vi "系统设置.vi"() -> ()   [LabVIEW 2016]
uses:
  <vilib>/Utility/miscctls.llb/LVPointTypeDef.ctl
  <vilib>/ptbypt/NI_PtbyPt.lvlib
  <vilib>/Utility/config.llb/NI_LVConfig.lvlib
  PLC/PLC.lvlib
panel:
  in  "updateconfiguration":T1={"主机"="27.154.58.30", "用户"="update", "密码"="std23506", "远程路径"="数据传输系统\\平台数据传输系统.exe", "下载文件名"="平台数据传输系统.exe", "软件版本"=""}
  in  "周期运行启动参数":T2
  in  "超标浓度报警":bool
  in  "更新":bool
  in  "模块启用配置":bool
  in  "短信报警设置":bool
  in  "首页显示设置":bool
  in  "跨度核查":bool
  in  "空白核查":bool
  out "选项卡控件":enum32{"自由设定", "国标协议", "流量设定"}(tab)
  in  "24H周期设置":bool[](xcontrol)
  in  "运行间隔":i16=4 min=1 max=24
  in  "流量阈值":dbl=4.0 min=1.0 max=24.0
  in  "时间阈值":u16=4 min=1 max=24
  in  "周期设置":enum16{"自由设定", "国标协议", "流量设定"}(ring)
  out "x = y?":bool
  in  "质控启动日期":string(combo)="关闭"
  in  "跨度核查时间":T3(ring)=enum."06H"
  in  "空白核查时间":T3(ring)=enum."02H"
  in  "输入密码":dbl
  out "布尔":bool
  in  "副屏显示设置":bool
  in  "开机启动":bool caption="氨氮禁用"
  in  "运行模式":enum16{"维护模式", "常规模式", "应急模式", "质控模式"}(ring)
  # "注：周期设置分为自由设定和国标协议两种。\n1：选择自由设定情况下：运行间隔将不可选用并变灰色，周期设置可自由手动勾选\n2：选择国标协议情况下：周期时间将由运行间隔选择的时间决定，下方周期设置被禁用并无法手动勾选。\n3：选择流量设定情况下：瞬时流量连续超过流量阈值到达时间阈值设定值，仪器将自动开启测量。"
  # "质控频次："
  # "零点核查时间："
  # "跨度核查时间："
  # "启动周期设置"
  # "m3/S"
  # "秒"
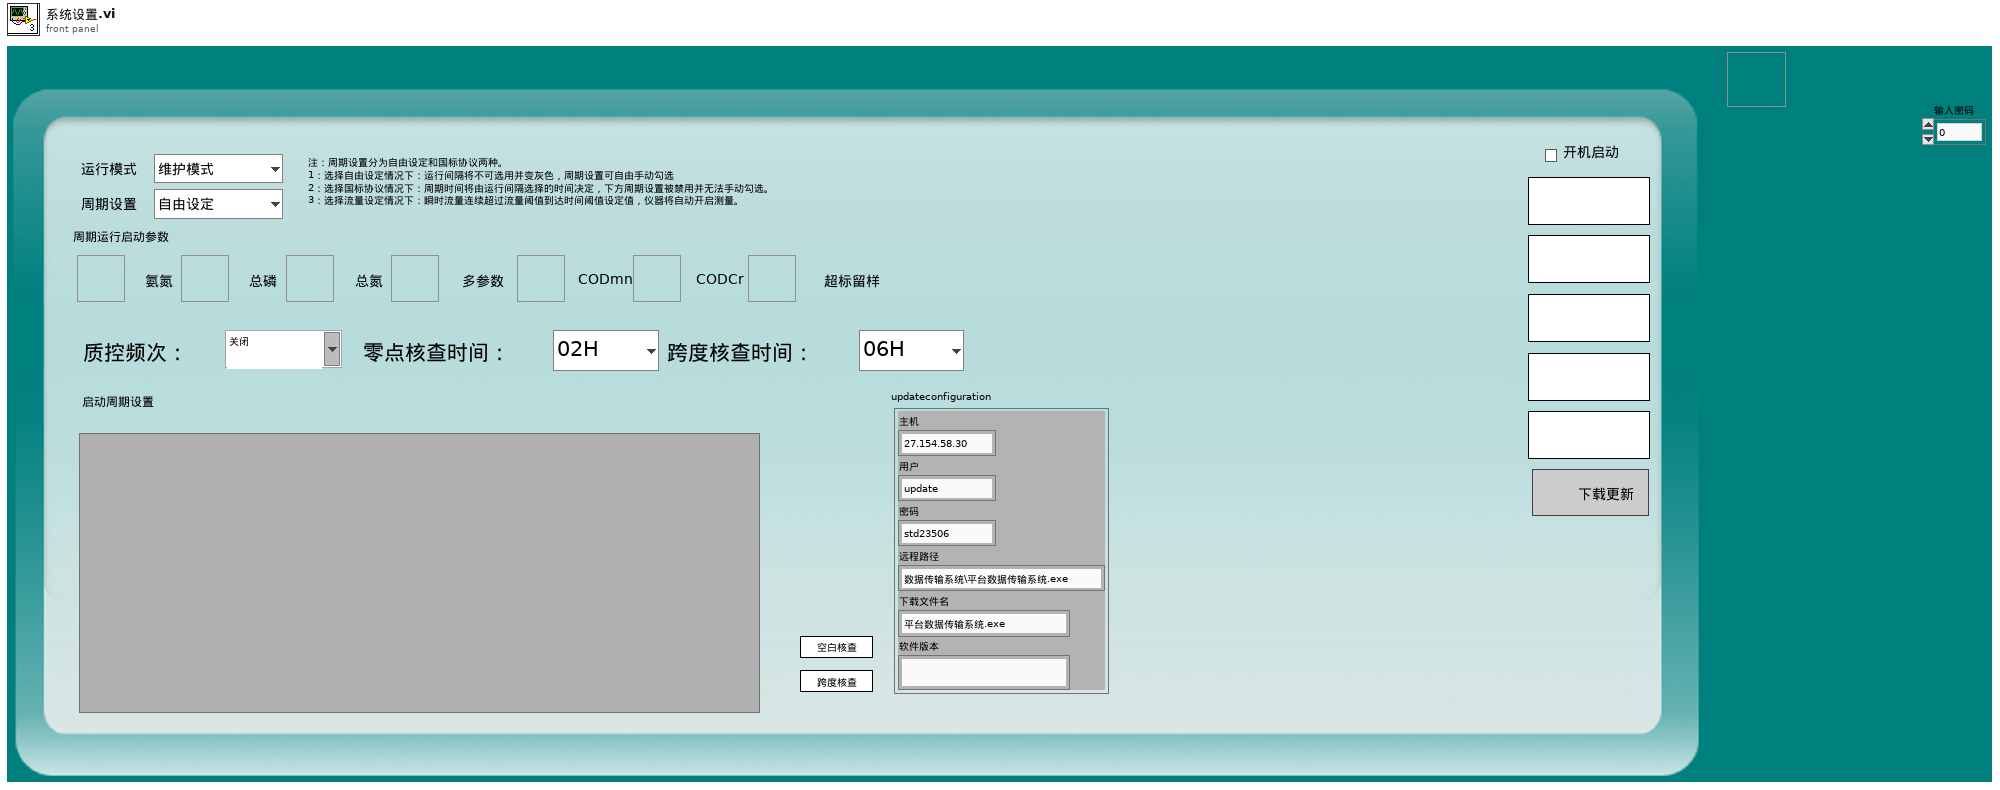
[diagram p1: front panel]
types:
  T1 = cluster{"主机":string, "用户":string, "密码":string, "远程路径":string, "下载文件名":string, "软件版本":string}
  T2 = cluster{"氨氮":bool, "总磷":bool, "总氮":bool, "多参数":bool, "CODmn":bool, "CODCr":bool, "超标留样":bool}
  T3 = enum16{"00H", "01H", "02H", "03H", "04H", "05H", "06H", "07H", "08H", "09H", "10H", "11H", "12H", "13H", "14H", "15H", "16H", "17H", "18H", "19H", "20H", "21H", "22H", "23H", "关闭"}
  T4 = typedef "NI_LVConfig.lvlib/Config Data RefNum.ctl" = refnum<k1>
  T5 = typedef "LVPointTypeDef.ctl" = cluster{"Horizontal":i16, "Vertical":i16}
  T6 = enum32{"Bad", "Idle", "Run top level", "Running"}
  T7 = enum32{"Invalid", "Standard", "Closed", "Hidden", "Minimized", "Maximized"}
  T8 = cluster{"运行模式":enum16{"维护模式", "常规模式", "应急模式", "质控模式"}}
  T9 = enum16{"启动测量", "标样核查", "零点核查", "跨度核查", "空白测试", "平行样测试", "加标回收", "空白校准", "标样校准", "初始化（清洗）", "停止测试", "仪器重启", "校时", "模式设置", "测量间隔设置"}
  T10 = cluster{"测量模式":enum16{"水样测量", "标样核查", "零点核查", "跨度核查", "空白测试", "加标回收", "平行样", "校零", "校标"}}
  T11 = cluster{"测试模式":enum16{"正常测试", "集成干预", "加标回收"}, "参数启用":cluster{"氨氮":bool, "总磷":bool, "总氮":bool, "多参数":bool, "CODMn":bool, "CODcr":bool, "超标留样":bool}}
  T12 = cluster{"运行模式":enum16{"维护模式", "常规模式", "应急模式", "质控模式"}, "质控频次":enum16{"关闭", "每天", "星期一", "星期二", "星期三", "星期四", "星期五", "星期六", "星期日"}, "空白核查时间":u16, "跨度核查时间":u16, "24H周期设置":bool[]}
  T13 = typedef "LVDateTimeRec.ctl" = cluster{"秒数的小数部分":dbl, "秒":i32, "分":i32, "时":i32, "日":i32, "月":i32, "年":i32, "天数（周）":i32, "天数（年）":i32, "DST":i32}
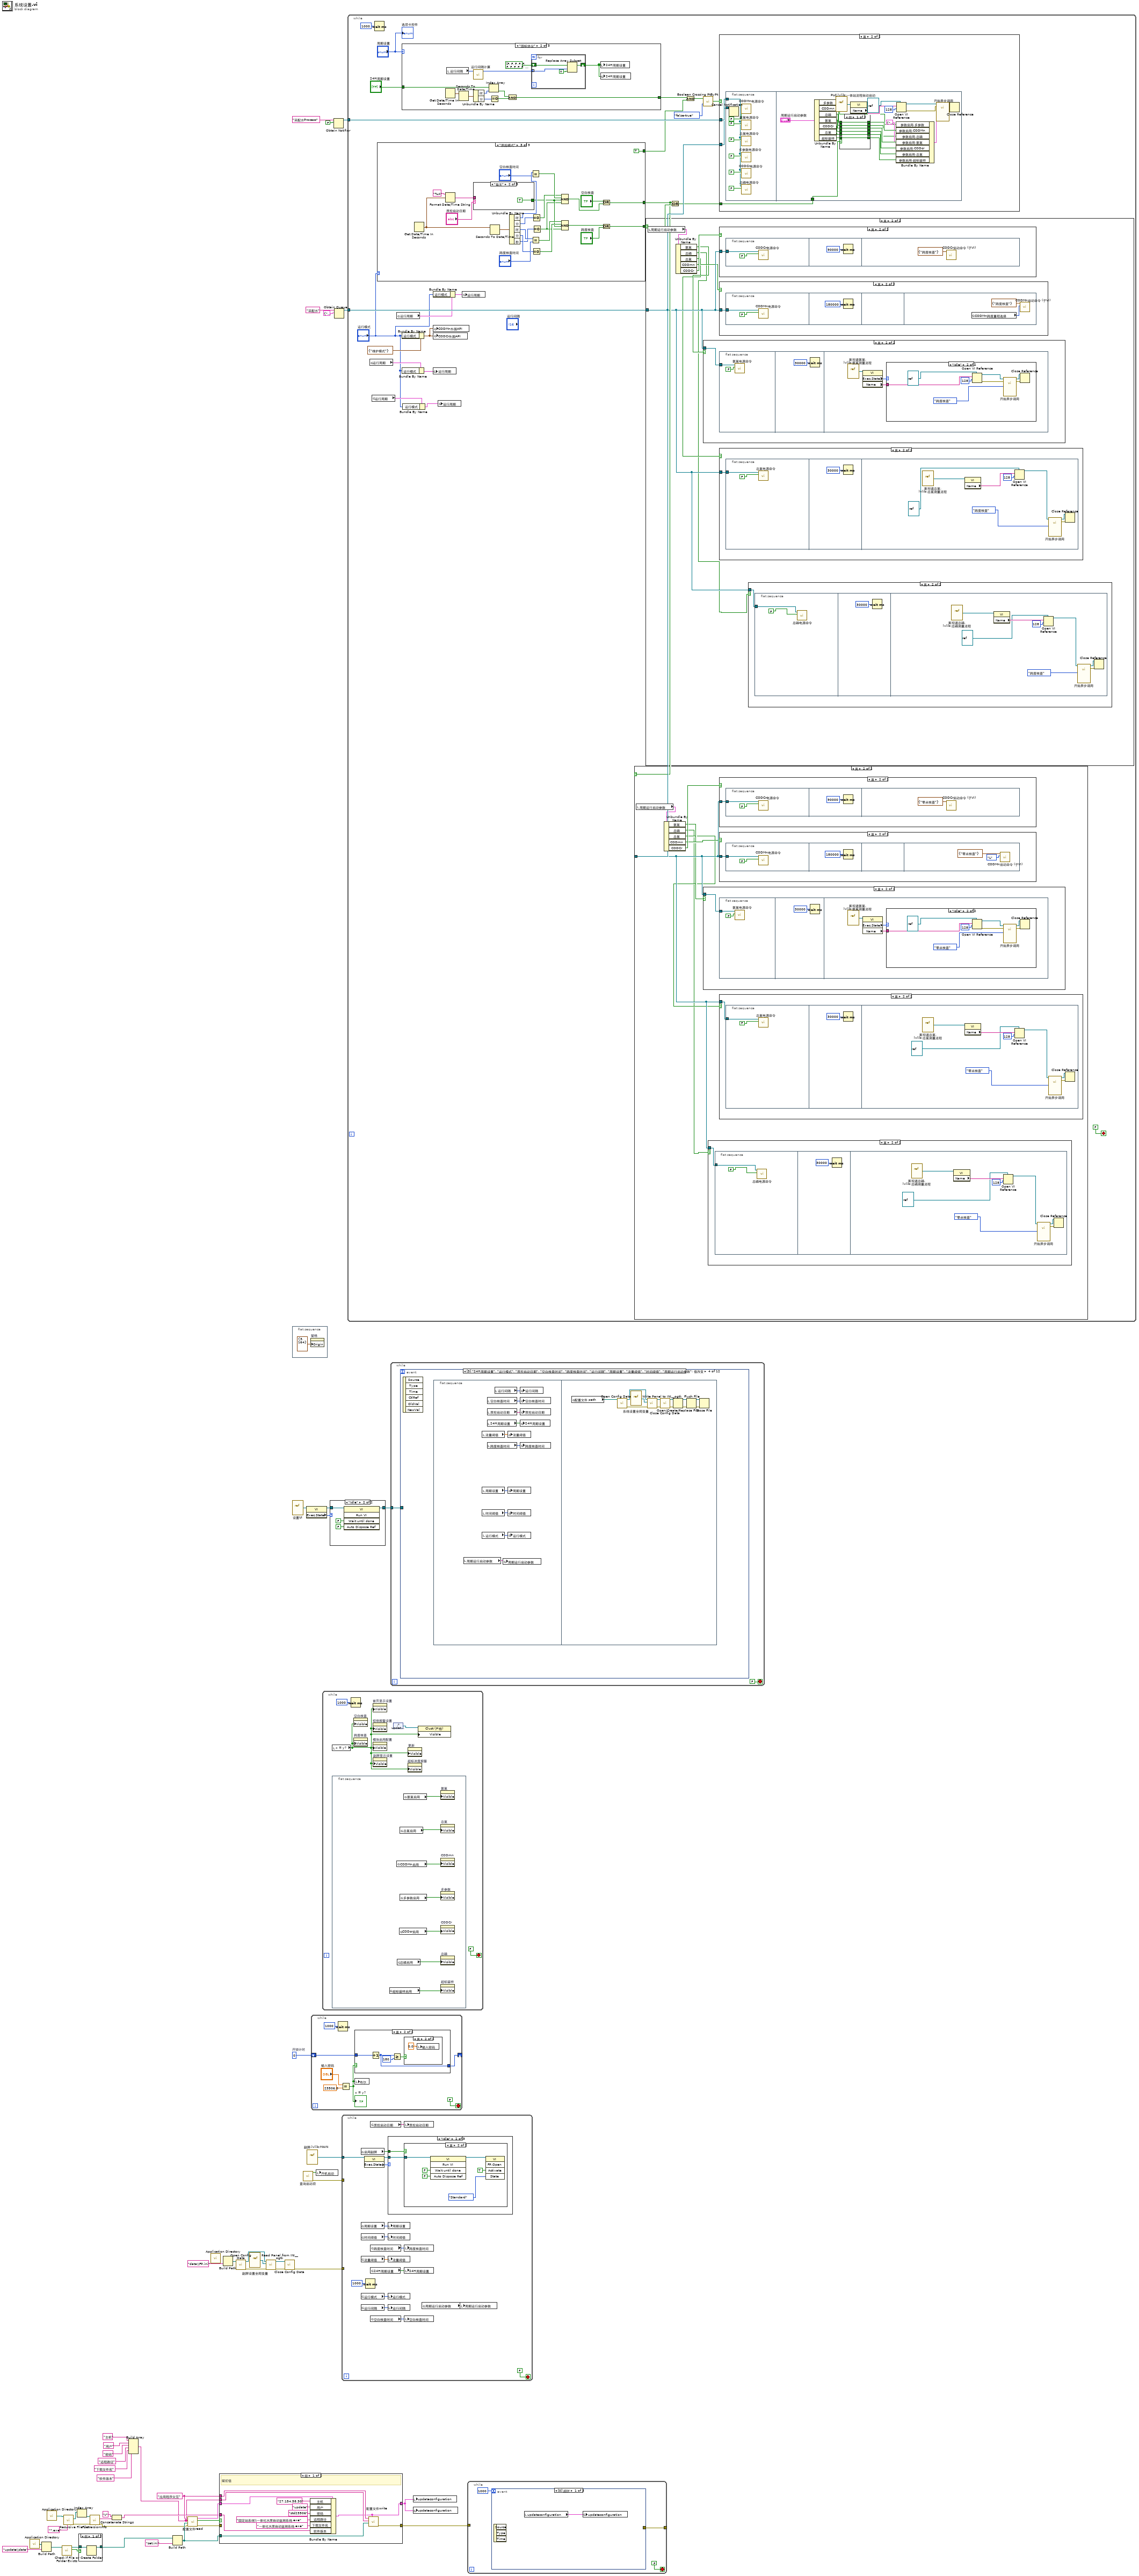
[diagram p0: block diagram]
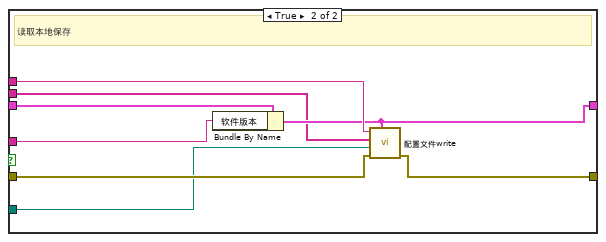
[diagram p3: hidden frame]
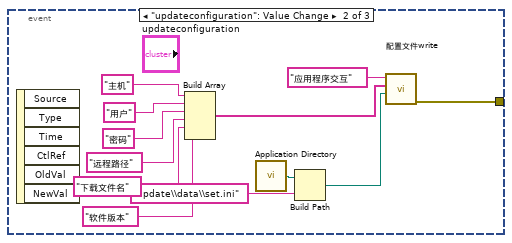
[diagram p4: hidden frame]
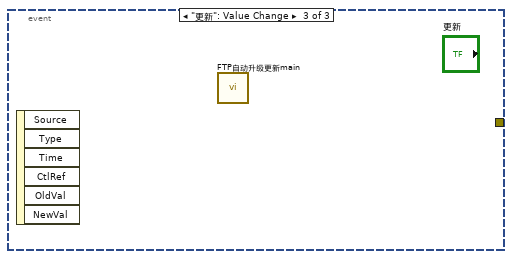
[diagram p5: hidden frame]
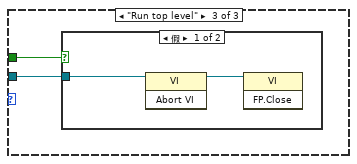
[diagram p11: hidden frame]
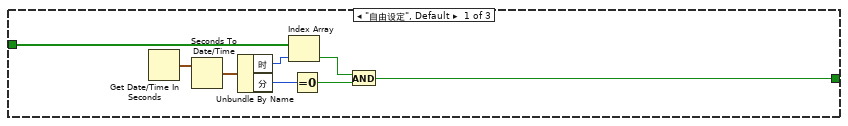
[diagram p13: hidden frame]
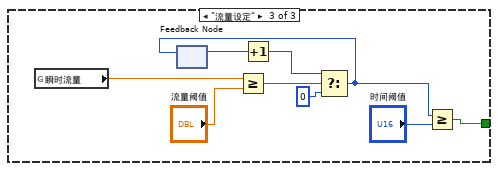
[diagram p14: hidden frame]
diagram:
  w28 = "应用程序交互" ("section")
  w48 = u32 0  # 开锁计时
  n1 = call <vilib>:"Application Directory.vi"() -> ("Application Directory"=w5:path)
  n2 = Build Path(base path=w5, name or relative path="update\\data" ("名称或相对路径")) -> (appended path=w6:path)
  n3 = call <vilib>:"Application Directory.vi"() -> ("Application Directory"=w23:path)
  n4 = call <vilib>:"Check if File or Folder Exists.vi"("path"=w6) -> ("file or folder exists?"=w7:bool, "dup path"=w8:path)  [unwired: 8 in, 1 out]
  n5 = call <vilib>:"Recursive File List.vi"("pattern"="*.exe", "Folder Path"=w23) -> ("error out"=w20:errorcluster, "All Files in Dir"=w22:path[])  [unwired: 5 in, 3 out]
  n6 = Index Array(array=w22) -> (element=w24:path)  [unwired: 1 in]
  n7 = case shown="假" w7 {
    tunnel: w8 -> [w54 w55]
    tunnel: [w53 w55] -> w3
    frame False {
      n8 = Create Folder(path (use dialog)=w54) -> (created path=w53:path)  [unwired: 2 in, 2 out]
    }
    frame True {
    }
  }
  n9 = call <vilib>:"FileVersionInfo.vi"("error in (no error)"=w20, "Application Path in"=w24) -> ("error out"=w17:errorcluster, "File Version Info"=w18:string)  [unwired: 6 in, 2 out]
  n10 = Concatenate Strings("V" ("字符串"), w18) -> (w16:string)
  n11 = Build Array("主机" ("section"), "用户" ("section"), "密码" ("key"), "远程路径" ("key"), "下载文件名" ("key"), "软件版本" ("key")) -> (w2:string[])
  n12 = Build Path(base path=w3, name or relative path="set.ini" ("名称或相对路径")) -> (appended path=w27:path)
  n13 = call "配置文件read.vi"("error in (no error)"=w17, "configuration file path"=w27, "键数组"=w2, "段"=w28) -> ("error out"=w26:errorcluster, "section exists?"=w29:bool, "updateconfiguration"=w25:T1)  [unwired: 5 in]
  n14 = call <vilib>:"Application Directory.vi"() -> ()  [unwired: 1 out]
  n15 = case shown="假" w29 {
    tunnel: w2 -> [w67 w71]
    tunnel: w28 -> [w66 w75]
    tunnel: w27 -> [w65 w69]
    tunnel: w26 -> [_ w70]
    tunnel: [w64 w68] -> w15
    tunnel: w25 -> [w58 w74]
    tunnel: [w56 w72] -> w1
    tunnel: w16 -> [w57 w73]
    frame False {
      # "赋初值"
      n16 = Bundle By Name(cluster=w58, "主机"="27.154.58.30" ("key"), "用户"="update", "密码"="std23506", "远程路径"="固定站系统\\一体化水质自动监测系统.exe", "下载文件名"="一体化水质自动监测系统.exe", "软件版本"=w57) -> (w56:T1)
      n17 = call "配置文件write.vi"("updateconfiguration"=w56, "configuration file path"=w65, "键数组"=w67, "段"=w66) -> ("error out"=w64:errorcluster)  [unwired: 7 in]
    }
    frame True {
      # "读取本地保存"
      n18 = Bundle By Name(cluster=w74, "软件版本"=w73) -> (w72:T1)
      n19 = call "配置文件write.vi"("updateconfiguration"=w72, "error in (no error)"=w70, "configuration file path"=w69, "键数组"=w71, "段"=w75) -> ("error out"=w68:errorcluster)  [unwired: 6 in]
    }
  }
  n20 = Build Path(name or relative path="data\\FP.ini" ("名称或相对路径")) -> (appended path=w37:path)  [unwired: 1 in]
  n21 = call <vilib>:"Open Config Data.vi"("configuration file path"=w37) -> ("error out"=w36:errorcluster, "refnum"=w33:T4)  [unwired: 8 in, 1 out]
  n22 = vi-ref "副屏设置全局变量.vi"() -> (w34:refnum<vi>)
  n23 = call <userlib>:"Read Panel from INI__ogtk.vi"("error in (no error)"=w36, "VI ref"=w34, "refnum"=w33) -> ("error out"=w35:errorcluster, "refnum out"=w32:T4)  [unwired: 7 in]
  n24 = call <vilib>:"Close Config Data.vi"("error in (no error)"=w35, "refnum"=w32) -> ("error out"=w31:errorcluster)  [unwired: 8 in, 1 out]
  n25 = flat-sequence {
    frame #0 {
      n26 = property on="窗格" class="Pane"("Origin"=T5 {"Horizontal"=3, "Vertical"=164} ("原点")) -> ()  [unwired: 2 in, 2 out]
    }
  }
  n27 = vi-ref "设置UI.vi"() -> (w43:refnum<vi>)
  n28 = call "查询启动项.vi"() -> ("error out"=w39:errorcluster, "包含启动项"=w49:bool)  [unwired: 9 in, 1 out]
  n29 = property class="VI"(reference=w43) -> (reference out=w41:refnum<vi>, "Exec.State"=w42:T6)  [unwired: 1 in, 1 out]
  n30 = vi-ref "副屏.lvlib:MAIN.vi"() -> (w44:refnum<vi>)
  n31 = while {
    shift-right: [w78] -> _
    shift-left: w48 -> [w79]
    stop <- FALSE stop-if-true
    n32 = Wait (ms)(milliseconds to wait=u32 1000 ("等待时间（毫秒）")) -> ()  [unwired: 1 out]
    n33 = Equal?(x="输入密码", y=23506.0) -> (x = y?=w77:bool)
    "x = y?" <- w77
    n34 = case shown="真" w77 {
      tunnel: w79 -> [_ w87]
      tunnel: [_ w86] -> w78
      frame False {
      }
      frame True {
        n35 = Increment(x=w87) -> (x+1=w86:u32)
        n36 = Greater Or Equal?(x=w86, y=u32 180) -> (x >= y?=w84:bool)
        n37 = case shown="真" w84 {
          frame False {
          }
          frame True {
            n38 = local write "输入密码"(0.0 ("输入密码")) -> ()
          }
        }
      }
    }
    n39 = local write "布尔"(w77) -> ()
  }
  n40 = local write "开机启动"(w49) -> ()
  n41 = while {
    stop <- FALSE stop-if-true
    n42 = local read "x = y?"() -> (w90:bool)
    n43 = flat-sequence {
      frame #0 {
        n44 = global read "系统设置全局变量.vi" "超标留样启用"() -> (w93:bool)
        n45 = global read "系统设置全局变量.vi" "CODMn启用"() -> (w97:bool)
        n46 = global read "系统设置全局变量.vi" "总磷启用"() -> (w94:bool)
        n47 = global read "系统设置全局变量.vi" "CODcr启用"() -> (w95:bool)
        n48 = global read "系统设置全局变量.vi" "总氮启用"() -> (w98:bool)
        n49 = global read "系统设置全局变量.vi" "多参数启用"() -> (w96:bool)
        n50 = global read "系统设置全局变量.vi" "氨氮启用"() -> (w99:bool)
        n51 = property on="氨氮" class="Bool (严格)"("Visible"=w99) -> ()  [unwired: 2 in, 2 out]
        n52 = property on="总氮" class="Bool (严格)"("Visible"=w98) -> ()  [unwired: 2 in, 2 out]
        n53 = property on="CODmn" class="Bool (严格)"("Visible"=w97) -> ()  [unwired: 2 in, 2 out]
        n54 = property on="多参数" class="Bool (严格)"("Visible"=w96) -> ()  [unwired: 2 in, 2 out]
        n55 = property on="CODCr" class="Bool (严格)"("Visible"=w95) -> ()  [unwired: 2 in, 2 out]
        n56 = property on="总磷" class="Bool (严格)"("Visible"=w94) -> ()  [unwired: 2 in, 2 out]
        n57 = property on="超标留样" class="Bool (严格)"("Visible"=w93) -> ()  [unwired: 2 in, 2 out]
      }
    }
    n58 = Wait (ms)(milliseconds to wait=u32 1000 ("等待时间（毫秒）")) -> ()  [unwired: 1 out]
    n59 = property on="空白核查" class="Bool"("Visible"=w90) -> ()  [unwired: 2 in, 2 out]
    n60 = property on="跨度核查" class="Bool"("Visible"=w90) -> ()  [unwired: 2 in, 2 out]
    n61 = property on="首页显示设置" class="Bool"("Visible"=w90) -> ()  [unwired: 2 in, 2 out]
    n62 = property on="短信报警设置" class="Bool"("Visible"=w90) -> ()  [unwired: 2 in, 2 out]
    n63 = property on="模块启用配置" class="Bool"("Visible"=w90) -> ()  [unwired: 2 in, 2 out]
    n64 = property on="副屏显示设置" class="Bool"("Visible"=w90) -> ()  [unwired: 2 in, 2 out]
    n65 = control-ref of="updateconfiguration"() -> (w89:refnum<vi>)
    n66 = property on="超标浓度报警" class="Bool"("Visible"=w90) -> ()  [unwired: 2 in, 2 out]
    n67 = property on="更新" class="Bool"("Visible"=w90) -> ()  [unwired: 2 in, 2 out]
    n68 = property class="Clust (严格)"(reference=w89, "Visible"=w90) -> ()  [unwired: 1 in, 2 out]
  }
  n69 = case shown="\"Idle\"" w42 {
    tunnel: w41 -> [w100 w104]
    tunnel: [w100 w103] -> w40
    frame "Bad", Default {
    }
    frame "Idle" {
      n70 = invoke class="VI" method="Run VI"(reference=w104, "Wait until done"=FALSE ("结束前等待"), "Auto Dispose Ref"=FALSE ("自动销毁引用")) -> (reference out=w103:refnum<vi>)  [unwired: 2 in, 4 out]
    }
  }
  n71 = Obtain Notifier(name (unnamed)="采配水Process" ("名称（未命名）"), notification data type=FALSE) -> (notifier out=w50:refnum<notifier>)  [unwired: 2 in, 2 out]
  n72 = Obtain Queue(name (unnamed)="采配水" ("名称（未命名）"), element data type=cluster{"命令":string, "数据":variant} {"命令"="", "数据"=variant}) -> (queue out=w45:refnum<queue>)  [unwired: 3 in, 2 out]
  n73 = while {
    tunnel: w44 -> [w117]
    tunnel: w39 -> [_]
    tunnel: w31 -> [_]
    stop <- FALSE stop-if-true
    n74 = global read "副屏设置全局变量.vi" "启用副屏"() -> (w115:bool)
    n75 = global read "系统设置全局变量.vi" "周期设置"() -> (w110:enum16{"自由设定", "国标协议", "流量设定"})
    n76 = global read "系统设置全局变量.vi" "时间阈值"() -> (w106:u16)
    n77 = global read "系统设置全局变量.vi" "流量阈值"() -> (w107:dbl)
    n78 = global read "系统设置全局变量.vi" "运行模式"() -> (w108:enum16{"维护模式", "常规模式", "应急模式", "质控模式"})
    n79 = global read "系统设置全局变量.vi" "运行间隔"() -> (w109:i16)
    n80 = property class="VI"(reference=w117) -> (reference out=w114:refnum<vi>, "Exec.State"=w116:T6)  [unwired: 1 in, 1 out]
    n81 = Wait (ms)(milliseconds to wait=u32 1000 ("等待时间（毫秒）")) -> ()  [unwired: 1 out]
    n82 = global read "系统设置全局变量.vi" "质控启动日期"() -> (w113:string)
    n83 = global read "系统设置全局变量.vi" "跨度核查时间"() -> (w111:u16)
    n84 = global read "系统设置全局变量.vi" "24H周期设置"() -> (w118:bool[])
    n85 = global read "系统设置全局变量.vi" "空白核查时间"() -> (w112:u16)
    n86 = case shown="\"Idle\"" w116 {
      tunnel: w115 -> [_ w121 w129]
      tunnel: w114 -> [_ w122 w130]
      frame "Bad", Default {
      }
      frame "Idle" {
        n87 = case shown="真" w121 {
          tunnel: w122 -> [_ w128]
          frame False {
          }
          frame True {
            n88 = invoke class="VI" method="Run VI"(reference=w128, "Wait until done"=FALSE ("结束前等待"), "Auto Dispose Ref"=FALSE ("自动销毁引用")) -> (reference out=w123:refnum<vi>)  [unwired: 2 in, 4 out]
            n89 = invoke class="VI" method="FP.Open"(reference=w123, "Activate"=TRUE ("激活？"), "State"=T7."Standard" ("状态")) -> ()  [unwired: 2 in, 5 out]
          }
        }
      }
      frame "Run top level" {
        n90 = case shown="假" w129 {
          tunnel: w130 -> [w131 _]
          frame False {
            n91 = invoke class="VI" method="Abort VI"(reference=w131) -> (reference out=w132:refnum<vi>)  [unwired: 2 in, 2 out]
            n92 = invoke class="VI" method="FP.Close"(reference=w132) -> ()  [unwired: 2 in, 3 out]
          }
          frame True {
          }
        }
      }
    }
    n93 = local write "周期设置"(w110) -> ()
    n94 = local write "时间阈值"(w106) -> ()
    n95 = local write "流量阈值"(w107) -> ()
    n96 = local write "运行模式"(w108) -> ()
    n97 = local write "运行间隔"(w109) -> ()
    n98 = local write "质控启动日期"(w113) -> ()
    n99 = local write "跨度核查时间"(w111) -> ()
    n100 = local write "24H周期设置"(w118) -> ()
    n101 = local write "空白核查时间"(w112) -> ()
    n102 = global read "系统设置全局变量.vi" "周期运行启动参数"() -> (w105:T2)
    n103 = local write "周期运行启动参数"(w105) -> ()
  }
  n104 = while {
    tunnel: w50 -> [w153]
    tunnel: w45 -> [w149]
    stop <- FALSE stop-if-true
    n105 = global read "总氮断电保存全局变量.vi" "运行周期"() -> (w137:T12)
    n106 = global read "总磷断电保存全局变量.vi" "运行周期"() -> (w135:T12)
    n107 = Wait (ms)(milliseconds to wait=u32 1000 ("等待时间（毫秒）")) -> ()  [unwired: 1 out]
    n108 = case shown="\"质控模式\"" "运行模式" {
      tunnel: [_ _ w346] -> w142
      tunnel: [_ _ w350] -> w141
      tunnel: [_ TRUE TRUE] -> w146
      frame "维护模式", Default {
      }
      frame "常规模式" {
      }
      frame "质控模式" {
        n109 = Get Date/Time In Seconds() -> (seconds since 1Jan1904=w357:timestamp)
        n110 = Format Date/Time String(time format string (%c)="%A" ("时间格式字符串(%c)"), seconds (now)=w357) -> (date/time string=w355:string)  [unwired: 1 in]
        n111 = case shown="\"每天\"" "质控启动日期" {
          selector: "质控启动日期" -> [w373 _ _]
          tunnel: [w372 TRUE FALSE] -> w358
          tunnel: w355 -> [w371 _ _]
          frame "星期二", "星期六", "星期日", "星期三", "星期四", "星期五", "星期一" {
            n112 = Equal?(x=w371, y=w373) -> (x = y?=w372:bool)
          }
          frame "每天" {
          }
          frame "关闭", Default {
          }
        }
        n113 = Seconds To Date/Time(time stamp (now)=w357) -> (date time rec=w370:T13)  [unwired: 1 in]
        n114 = Unbundle By Name(w370) -> ("时"=w369:i32, "分"=w367:i32, "时"=w363:i32, "分"=w362:i32, "秒"=w354:i32)
        n115 = Equal?(x=w369, y="空白核查时间") -> (x = y?=w366:bool)
        n116 = Equal?(x=w363, y="跨度核查时间") -> (x = y?=w361:bool)
        n117 = Equal To 0?(x=w367) -> (x = 0?=w365:bool)
        n118 = Equal To 0?(x=w362) -> (x = 0?=w360:bool)
        n119 = Equal To 0?(x=w354) -> (x = 0?=w353:bool)
        n120 = Compound Arithmetic op=AND ("复合运算")(w365, w366, w358, w353) -> (w351:bool)
        n121 = Compound Arithmetic op=AND ("复合运算")(w361, w360, w358, w353) -> (w348:bool)
        n122 = Or(x="空白核查", y=w351) -> (x .or. y?=w350:bool)
        n123 = Or(x=w348, y="跨度核查") -> (x .or. y?=w346:bool)
      }
    }
    n124 = global read "氨氮断电保存全局变量.vi" "运行周期"() -> (w139:T12)
    n125 = case shown="\"国标协议\"" "周期设置" {
      tunnel: [w157 w164 w180] -> w145
      tunnel: "24H周期设置" -> [w156 w165 _]
      frame "自由设定", Default {
        n126 = Get Date/Time In Seconds() -> (seconds since 1Jan1904=w158:timestamp)
        n127 = Seconds To Date/Time(time stamp (now)=w158) -> (date time rec=w159:T13)  [unwired: 1 in]
        n128 = Unbundle By Name(w159) -> ("时"=w162:i32, "分"=w160:i32)
        n129 = Index Array(array=w156, index=w162) -> (element=w163:bool)
        n130 = Equal To 0?(x=w160) -> (x = 0?=w161:bool)
        n131 = And(x=w163, y=w161) -> (x .and. y?=w157:bool)
      }
      frame "国标协议" {
        n132 = Get Date/Time In Seconds() -> (seconds since 1Jan1904=w166:timestamp)
        n133 = local read "运行间隔"() -> (w175:i16)
        n134 = Seconds To Date/Time(time stamp (now)=w166) -> (date time rec=w167:T13)  [unwired: 1 in]
        n135 = call "运行间隔计算.vi"("运行周期"=w175) -> ("数组"=w174:i32[])  [unwired: 10 in]
        n136 = Unbundle By Name(w167) -> ("时"=w170:i32, "分"=w168:i32)
        n137 = Index Array(array=w165, index=w170) -> (element=w171:bool)
        n138 = Equal To 0?(x=w168) -> (x = 0?=w169:bool)
        n139 = And(x=w171, y=w169) -> (x .and. y?=w164:bool)
        n140 = for {
          tunnel: w174 -> [w178] mode=indexing
          shift-right: [w176] -> w172
          shift-left: bool[] [FALSE, FALSE, FALSE, FALSE, FALSE, FALSE, FALSE, FALSE, FALSE, FALSE, FALSE, FALSE, FALSE, FALSE, FALSE, FALSE, FALSE, FALSE, FALSE, FALSE, FALSE, FALSE, FALSE, FALSE] ("24H周期设置") -> [w179]
          n141 = Replace Array Subset(array=w179, new element=TRUE ("新元素/子数组"), index=w178) -> (w176:bool[])
        }
        n142 = local write "24H周期设置"(w172) -> ()
        n143 = global write "系统设置全局变量.vi" "24H周期设置"(w172) -> ()
      }
      frame "流量设定" {
        n144 = global read "流量计全局变量.vi" "瞬时流量"() -> (w188:dbl)
        n145 = feedback #1() -> (w185:i16)  [unwired: 1 in]
        n146 = Greater Or Equal?(x=w188, y="流量阈值") -> (x >= y?=w183:bool)
        n147 = Increment(x=w185) -> (x+1=w184:i16)
        n148 = Select(t=w184, s=w183, f=i16 0) -> (s? t:f=w182:i16)
        n149 = feedback-in #1(w182) -> ()
        n150 = Greater Or Equal?(x=w182, y="时间阈值") -> (x >= y?=w180:bool)
      }
    }
    n151 = Bundle By Name(cluster=T8 {"运行模式"=enum."维护模式"} ("外围API"), "运行模式"="运行模式") -> (w143:T8)
    n152 = Bundle By Name(cluster=w137, "运行模式"="运行模式") -> (w136:T12)
    n153 = Bundle By Name(cluster=w135, "运行模式"="运行模式") -> (w134:T12)
    n154 = Bundle By Name(cluster=w139, "运行模式"="运行模式") -> (w138:T12)
    n155 = global write "总氮断电保存全局变量.vi" "运行周期"(w136) -> ()
    n156 = global write "CODMN外部API.vi" "CODMn外围API"(w143) -> ()
    n157 = global write "CODCr外部API.vi" "CODCr外围API"(w143) -> ()
    n158 = global write "总磷断电保存全局变量.vi" "运行周期"(w134) -> ()
    n159 = global write "氨氮断电保存全局变量.vi" "运行周期"(w138) -> ()
    n160 = case shown="真" w141 {
      tunnel: w149 -> [_ w252]
      frame False {
      }
      frame True {
        n161 = local read "周期运行启动参数"() -> (w251:T2)
        n162 = Unbundle By Name(w251) -> ("氨氮"=w248:bool, "总磷"=w246:bool, "总氮"=w247:bool, "CODmn"=w249:bool, "CODCr"=w250:bool)
        n163 = case shown="真" w248 {
          tunnel: w252 -> [_ w288]
          frame False {
          }
          frame True {
            n164 = flat-sequence {
              tunnel: w288 -> [w289]
              frame #0 {
                n165 = call "氨氮电源命令.vi"("通电/断电"=FALSE, "队列"=w289) -> ()  [unwired: 9 in, 1 out]
              }
              frame #1 {
                n166 = Wait (ms)(milliseconds to wait=u32 30000 ("等待时间（毫秒）")) -> ()  [unwired: 1 out]
              }
              frame #2 {
                n167 = vi-ref "斯坦道氨氮.lvlib:氨氮测量流程.vi"() -> (w294:refnum<vi>)
                n168 = property class="VI"(reference=w294) -> ("Exec.State"=w292:T6, "Name"=w293:string)  [unwired: 1 in, 2 out]
                n169 = case shown="\"Idle\"" w292 {
                  tunnel: w293 -> [_ w299]
                  frame "Bad", Default {
                  }
                  frame "Idle" {
                    n170 = Open VI Reference(type specifier VI Refnum (for type only)=refnum<vi> refnum, vi path=w299, options=128 ("选项")) -> (vi reference=w297:refnum<vi>, error out=w300:errorcluster)  [unwired: 3 in]
                    n171 = call-by-ref "开始异步调用"(reference=w297, error in=w300, "控制命令"=T9."零点核查") -> (reference out=w301:refnum<vi>, error out=w302:errorcluster)  [unwired: 11 in]
                    n172 = Close Reference(reference=w301, error in (no error)=w302) -> ()  [unwired: 1 out]
                  }
                }
              }
            }
          }
        }
        n173 = case shown="真" w246 {
          tunnel: w252 -> [_ w253]
          frame False {
          }
          frame True {
            n174 = flat-sequence {
              tunnel: w253 -> [w255]
              frame #0 {
                n175 = call "总磷电源命令.vi"("通电/断电"=FALSE, "队列"=w255) -> ()  [unwired: 9 in, 1 out]
              }
              frame #1 {
                n176 = Wait (ms)(milliseconds to wait=u32 30000 ("等待时间（毫秒）")) -> ()  [unwired: 1 out]
              }
              frame #2 {
                n177 = vi-ref "斯坦道总磷.lvlib:总磷测量流程.vi"() -> (w262:refnum<vi>)
                n178 = property class="VI"(reference=w262) -> ("Name"=w263:string)  [unwired: 1 in, 2 out]
                n179 = Open VI Reference(type specifier VI Refnum (for type only)=refnum<vi> refnum, vi path=w263, options=128 ("选项")) -> (vi reference=w261:refnum<vi>)  [unwired: 3 in, 1 out]
                n180 = call-by-ref "开始异步调用"(reference=w261, "控制命令"=T9."零点核查") -> (reference out=w260:refnum<vi>, error out=w259:errorcluster)  [unwired: 12 in]
                n181 = Close Reference(reference=w260, error in (no error)=w259) -> ()  [unwired: 1 out]
              }
            }
          }
        }
        n182 = case shown="真" w250 {
          tunnel: w252 -> [_ w265]
          frame False {
          }
          frame True {
            n183 = flat-sequence {
              tunnel: w265 -> [w266]
              frame #0 {
                n184 = call "CODCr电源命令.vi"("通电/断电"=FALSE, "队列"=w266) -> ()  [unwired: 9 in, 1 out]
              }
              frame #1 {
                n185 = Wait (ms)(milliseconds to wait=u32 90000 ("等待时间（毫秒）")) -> ()  [unwired: 1 out]
              }
              frame #2 {
                n186 = call "CODCr启动命令 (子VI).vi"("启动测量模式"=T10 {"测量模式"=enum."零点核查"}) -> ()  [unwired: 11 in]
              }
            }
          }
        }
        n187 = case shown="真" w249 {
          tunnel: w252 -> [_ w270]
          frame False {
          }
          frame True {
            n188 = flat-sequence {
              tunnel: w270 -> [w271]
              frame #0 {
                n189 = call "CODMn电源命令.vi"("通电/断电"=FALSE, "队列"=w271) -> ()  [unwired: 9 in, 1 out]
              }
              frame #1 {
                n190 = Wait (ms)(milliseconds to wait=u32 180000 ("等待时间（毫秒）")) -> ()  [unwired: 1 out]
              }
              frame #2 {
              }
              frame #3 {
                n191 = call "CODMn启动命令 (子VI).vi"("CODMn量程切换"=enum32{"H", "L", "AUTO"}."L", "启动测量模式"=T10 {"测量模式"=enum."零点核查"}) -> ()  [unwired: 10 in]
              }
            }
          }
        }
        n192 = case shown="真" w247 {
          tunnel: w252 -> [_ w276]
          frame False {
          }
          frame True {
            n193 = flat-sequence {
              tunnel: w276 -> [w278]
              frame #0 {
                n194 = call "总氮电源命令.vi"("通电/断电"=FALSE, "队列"=w278) -> ()  [unwired: 9 in, 1 out]
              }
              frame #1 {
                n195 = Wait (ms)(milliseconds to wait=u32 30000 ("等待时间（毫秒）")) -> ()  [unwired: 1 out]
              }
              frame #2 {
                n196 = vi-ref "斯坦道总氮.lvlib:总氮测量流程.vi"() -> (w285:refnum<vi>)
                n197 = property class="VI"(reference=w285) -> ("Name"=w286:string)  [unwired: 1 in, 2 out]
                n198 = Open VI Reference(type specifier VI Refnum (for type only)=refnum<vi> refnum, vi path=w286, options=128 ("选项")) -> (vi reference=w284:refnum<vi>)  [unwired: 3 in, 1 out]
                n199 = call-by-ref "开始异步调用"(reference=w284, "控制命令"=T9."零点核查") -> (reference out=w283:refnum<vi>, error out=w282:errorcluster)  [unwired: 12 in]
                n200 = Close Reference(reference=w283, error in (no error)=w282) -> ()  [unwired: 1 out]
              }
            }
          }
        }
      }
    }
    n201 = case shown="真" w142 {
      tunnel: w149 -> [_ w195]
      frame False {
      }
      frame True {
        n202 = local read "周期运行启动参数"() -> (w194:T2)
        n203 = Unbundle By Name(w194) -> ("氨氮"=w191:bool, "总磷"=w189:bool, "总氮"=w190:bool, "CODmn"=w192:bool, "CODCr"=w193:bool)
        n204 = case shown="真" w191 {
          tunnel: w195 -> [_ w231]
          frame False {
          }
          frame True {
            n205 = flat-sequence {
              tunnel: w231 -> [w232]
              frame #0 {
                n206 = call "氨氮电源命令.vi"("通电/断电"=FALSE, "队列"=w232) -> ()  [unwired: 9 in, 1 out]
              }
              frame #1 {
                n207 = Wait (ms)(milliseconds to wait=u32 30000 ("等待时间（毫秒）")) -> ()  [unwired: 1 out]
              }
              frame #2 {
                n208 = vi-ref "斯坦道氨氮.lvlib:氨氮测量流程.vi"() -> (w237:refnum<vi>)
                n209 = property class="VI"(reference=w237) -> ("Exec.State"=w235:T6, "Name"=w236:string)  [unwired: 1 in, 2 out]
                n210 = case shown="\"Idle\"" w235 {
                  tunnel: w236 -> [_ w242]
                  frame "Bad", Default {
                  }
                  frame "Idle" {
                    n211 = Open VI Reference(type specifier VI Refnum (for type only)=refnum<vi> refnum, vi path=w242, options=128 ("选项")) -> (vi reference=w240:refnum<vi>, error out=w243:errorcluster)  [unwired: 3 in]
                    n212 = call-by-ref "开始异步调用"(reference=w240, error in=w243, "控制命令"=T9."跨度核查") -> (reference out=w244:refnum<vi>, error out=w245:errorcluster)  [unwired: 11 in]
                    n213 = Close Reference(reference=w244, error in (no error)=w245) -> ()  [unwired: 1 out]
                  }
                }
              }
            }
          }
        }
        n214 = case shown="真" w193 {
          tunnel: w195 -> [_ w208]
          frame False {
          }
          frame True {
            n215 = flat-sequence {
              tunnel: w208 -> [w209]
              frame #0 {
                n216 = call "CODCr电源命令.vi"("通电/断电"=FALSE, "队列"=w209) -> ()  [unwired: 9 in, 1 out]
              }
              frame #1 {
                n217 = Wait (ms)(milliseconds to wait=u32 90000 ("等待时间（毫秒）")) -> ()  [unwired: 1 out]
              }
              frame #2 {
                n218 = call "CODCr启动命令 (子VI).vi"("启动测量模式"=T10 {"测量模式"=enum."跨度核查"}) -> ()  [unwired: 11 in]
              }
            }
          }
        }
        n219 = case shown="真" w192 {
          tunnel: w195 -> [_ w213]
          frame False {
          }
          frame True {
            n220 = flat-sequence {
              tunnel: w213 -> [w214]
              frame #0 {
                n221 = call "CODMn电源命令.vi"("通电/断电"=FALSE, "队列"=w214) -> ()  [unwired: 9 in, 1 out]
              }
              frame #1 {
                n222 = Wait (ms)(milliseconds to wait=u32 180000 ("等待时间（毫秒）")) -> ()  [unwired: 1 out]
              }
              frame #2 {
              }
              frame #3 {
                n223 = global read "CODMn断电保存全局变量.vi" "CODMn跨度量程选择"() -> (w217:enum32{"H", "L", "AUTO"})
                n224 = call "CODMn启动命令 (子VI).vi"("CODMn量程切换"=w217, "启动测量模式"=T10 {"测量模式"=enum."跨度核查"}) -> ()  [unwired: 10 in]
              }
            }
          }
        }
        n225 = case shown="真" w190 {
          tunnel: w195 -> [_ w219]
          frame False {
          }
          frame True {
            n226 = flat-sequence {
              tunnel: w219 -> [w221]
              frame #0 {
                n227 = call "总氮电源命令.vi"("通电/断电"=FALSE, "队列"=w221) -> ()  [unwired: 9 in, 1 out]
              }
              frame #1 {
                n228 = Wait (ms)(milliseconds to wait=u32 30000 ("等待时间（毫秒）")) -> ()  [unwired: 1 out]
              }
              frame #2 {
                n229 = vi-ref "斯坦道总氮.lvlib:总氮测量流程.vi"() -> (w228:refnum<vi>)
                n230 = property class="VI"(reference=w228) -> ("Name"=w229:string)  [unwired: 1 in, 2 out]
                n231 = Open VI Reference(type specifier VI Refnum (for type only)=refnum<vi> refnum, vi path=w229, options=128 ("选项")) -> (vi reference=w227:refnum<vi>)  [unwired: 3 in, 1 out]
                n232 = call-by-ref "开始异步调用"(reference=w227, "控制命令"=T9."跨度核查") -> (reference out=w226:refnum<vi>, error out=w225:errorcluster)  [unwired: 12 in]
                n233 = Close Reference(reference=w226, error in (no error)=w225) -> ()  [unwired: 1 out]
              }
            }
          }
        }
        n234 = case shown="真" w189 {
          tunnel: w195 -> [_ w196]
          frame False {
          }
          frame True {
            n235 = flat-sequence {
              tunnel: w196 -> [w198]
              frame #0 {
                n236 = call "总磷电源命令.vi"("通电/断电"=FALSE, "队列"=w198) -> ()  [unwired: 9 in, 1 out]
              }
              frame #1 {
                n237 = Wait (ms)(milliseconds to wait=u32 30000 ("等待时间（毫秒）")) -> ()  [unwired: 1 out]
              }
              frame #2 {
                n238 = vi-ref "斯坦道总磷.lvlib:总磷测量流程.vi"() -> (w205:refnum<vi>)
                n239 = property class="VI"(reference=w205) -> ("Name"=w206:string)  [unwired: 1 in, 2 out]
                n240 = Open VI Reference(type specifier VI Refnum (for type only)=refnum<vi> refnum, vi path=w206, options=128 ("选项")) -> (vi reference=w204:refnum<vi>)  [unwired: 3 in, 1 out]
                n241 = call-by-ref "开始异步调用"(reference=w204, "控制命令"=T9."跨度核查") -> (reference out=w203:refnum<vi>, error out=w202:errorcluster)  [unwired: 12 in]
                n242 = Close Reference(reference=w203, error in (no error)=w202) -> ()  [unwired: 1 out]
              }
            }
          }
        }
      }
    }
    n243 = Or(x=w141, y=w142) -> (x .or. y?=w140:bool)
    n244 = And(x=w145, y=w146) -> (x .and. y?=w144:bool)
    n245 = call <vilib>:"Boolean Crossing PtByPt.vi"("direction"=enum16{"either", "false-true", "true-false"}."false-true", "input"=w144) -> ("crossing"=w151:bool)  [unwired: 1 in]
    n246 = case shown="真" w151 {
      tunnel: w153 -> [_ w305]
      tunnel: w149 -> [_ w304]
      tunnel: w140 -> [_ w303]
      frame False {
      }
      frame True {
        n247 = flat-sequence {
          tunnel: w305 -> [w313]
          tunnel: w304 -> [w307]
          tunnel: w303 -> [w329]
          frame #0 {
            n248 = Cancel Notification(0:w313) -> ()  [unwired: 1 in, 3 out]
            n249 = call "CODMn电源命令.vi"("通电/断电"=FALSE, "队列"=w307) -> ()  [unwired: 9 in, 1 out]
            n250 = call "氨氮电源命令.vi"("通电/断电"=FALSE, "队列"=w307) -> ()  [unwired: 9 in, 1 out]
            n251 = call "总氮电源命令.vi"("通电/断电"=FALSE, "队列"=w307) -> ()  [unwired: 9 in, 1 out]
            n252 = call "多参数电源命令.vi"("通电/断电"=FALSE, "队列"=w307) -> ()  [unwired: 9 in, 1 out]
            n253 = call "CODCr电源命令.vi"("通电/断电"=FALSE, "队列"=w307) -> ()  [unwired: 9 in, 1 out]
            n254 = call "总磷电源命令.vi"("通电/断电"=FALSE, "队列"=w307) -> ()  [unwired: 9 in, 1 out]
          }
          frame #1 {
            n255 = Unbundle By Name("周期运行启动参数") -> ("多参数"=w324:bool, "CODmn"=w323:bool, "总磷"=w322:bool, "氨氮"=w321:bool, "CODCr"=w318:bool, "总氮"=w316:bool, "超标留样"=w314:bool)
            n256 = vi-ref "PLC.lvlib:一体站流程自动启动.vi"() -> (w334:refnum<vi>)
            n257 = case shown="假" w329 {
              tunnel: [w344 _] -> w338
              tunnel: [w343 _] -> w320
              tunnel: [w342 _] -> w337
              tunnel: w323 -> [w344 _]
              tunnel: w322 -> [w343 _]
              tunnel: w321 -> [w342 _]
              tunnel: [w341 _] -> w319
              tunnel: w318 -> [w341 _]
              tunnel: [w340 _] -> w317
              tunnel: w316 -> [w340 _]
              tunnel: [w339 _] -> w315
              tunnel: w314 -> [w339 _]
              frame False {
              }
              frame True {
              }
            }
            n258 = property class="VI"(reference=w334) -> ("Name"=w335:string)  [unwired: 1 in, 2 out]
            n259 = Bundle By Name(cluster=T11 {"测试模式"=enum."正常测试", "参数启用"={"氨氮"=FALSE, "总磷"=FALSE, "总氮"=FALSE, "多参数"=FALSE, "CODMn"=FALSE, "CODcr"=FALSE, "超标留样"=FALSE}} ("参数"), "参数启用.多参数"=w324, "参数启用.CODMn"=w338, "参数启用.总磷"=w320, "参数启用.氨氮"=w337, "参数启用.CODcr"=w319, "参数启用.总氮"=w317, "参数启用.超标留样"=w315) -> (w326:T11)
            n260 = Open VI Reference(type specifier VI Refnum (for type only)=refnum<vi> refnum, vi path=w335, options=128 ("选项")) -> (vi reference=w333:refnum<vi>, error out=w332:errorcluster)  [unwired: 3 in]
            n261 = call-by-ref "开始异步调用"(reference=w333, error in=w332, "参数"=w326) -> (reference out=w331:refnum<vi>, error out=w330:errorcluster)  [unwired: 11 in]
            n262 = Close Reference(reference=w331, error in (no error)=w330) -> ()  [unwired: 1 out]
          }
        }
      }
    }
    "选项卡控件" <- "周期设置"
  }
  n263 = while {
    tunnel: w40 -> [w376]
    stop <- FALSE stop-if-true
    n264 = event shown="[3] \"24H周期设置\", \"运行模式\", \"质控启动日期\", \"空白核查时间\", \"跨度核查时间\", \"运行间隔\", \"周期设置\", \"流量阈值\", \"时间阈值\", \"周期运行启动参数\": 值改变" {
      selector: _ -> [_ _ _ _ _ _ _ _ _ _ _ _]
      dyn-events: _ -> [_ _ _ _ _ _ _ _ _ _ _ _]
      timeout: _ -> [_ _ _ _ _ _ _ _ _ _ _ _]
      tunnel: w376 -> [_ _ _ _ _ _ _ _ _ _ w423 _]
      event Timeout {
        n265 = event-data() -> ()  [unwired: 1 in, 3 out]
      }
      event "模块启用配置": Value Change {
        n266 = event-data() -> ()  [unwired: 1 in, 6 out]
        n267 = call "模块启用配置框.vi"() -> ()  [unwired: 12 in]
      }
      event "超标浓度报警": Value Change {
        n268 = event-data() -> ()  [unwired: 1 in, 6 out]
        n269 = call "超标浓度报警配置.vi"() -> ()  [unwired: 12 in]
      }
      event "24H周期设置", "运行模式", "质控启动日期", "空白核查时间", "跨度核查时间", "运行间隔", "周期设置", "流量阈值", "时间阈值", "周期运行启动参数": Value Change {
        n270 = event-data() -> ()  [unwired: 1 in, 6 out]
        n271 = flat-sequence {
          frame #0 {
            n272 = local read "周期运行启动参数"() -> (w378:T2)
            n273 = local read "流量阈值"() -> (w379:dbl)
            n274 = local read "周期设置"() -> (w381:enum16{"自由设定", "国标协议", "流量设定"})
            n275 = local read "时间阈值"() -> (w380:u16)
            n276 = local read "运行模式"() -> (w387:enum16{"维护模式", "常规模式", "应急模式", "质控模式"})
            n277 = local read "空白核查时间"() -> (w384:T3)
            n278 = local read "质控启动日期"() -> (w385:string)
            n279 = local read "24H周期设置"() -> (w386:bool[])
            n280 = local read "跨度核查时间"() -> (w383:T3)
            n281 = local read "运行间隔"() -> (w382:i16)
            n282 = global write "系统设置全局变量.vi" "周期运行启动参数"(w378) -> ()
            n283 = global write "系统设置全局变量.vi" "流量阈值"(w379) -> ()
            n284 = global write "系统设置全局变量.vi" "周期设置"(w381) -> ()
            n285 = global write "系统设置全局变量.vi" "时间阈值"(w380) -> ()
            n286 = global write "系统设置全局变量.vi" "运行模式"(w387) -> ()
            n287 = global write "系统设置全局变量.vi" "运行间隔"(w382) -> ()
            n288 = global write "系统设置全局变量.vi" "空白核查时间"(w384) -> ()
            n289 = global write "系统设置全局变量.vi" "质控启动日期"(w385) -> ()
            n290 = global write "系统设置全局变量.vi" "24H周期设置"(w386) -> ()
            n291 = global write "系统设置全局变量.vi" "跨度核查时间"(w383) -> ()
          }
          frame #1 {
            n292 = global read "ping全局.vi" "配置文件 path"() -> (w388:path)
            n293 = call <vilib>:"Open Config Data.vi"("configuration file path"=w388) -> ("error out"=w396:errorcluster, "refnum"=w399:T4)  [unwired: 8 in, 1 out]
            n294 = vi-ref "系统设置全局变量.vi"() -> (w398:refnum<vi>)
            n295 = call <userlib>:"Write Panel to INI__ogtk.vi"("error in (no error)"=w396, "VI ref"=w398, "refnum"=w399) -> ("error out"=w395:errorcluster, "refnum out"=w397:T4)  [unwired: 7 in]
            n296 = call <vilib>:"Close Config Data.vi"("error in (no error)"=w395, "refnum"=w397) -> ("error out"=w390:errorcluster, "file path"=w389:path)  [unwired: 8 in]
            n297 = Open/Create/Replace File(file path (use dialog)=w389, error in=w390) -> (refnum out=w393:refnum<file>, error out=w394:errorcluster)  [unwired: 4 in, 1 out]
            n298 = Flush File(refnum=w393, error in=w394) -> (refnum out=w392:refnum<file>, error out=w391:errorcluster)
            n299 = Close File(refnum=w392, error in=w391) -> ()  [unwired: 2 out]
          }
        }
      }
      event "运行间隔": Mouse Down {
        n300 = event-data() -> ("CtlRef"=w403:refnum<vi>)  [unwired: 1 in, 7 out]
        n301 = property class="DigNum (严格)"(reference=w403) -> (reference out=w402:refnum<vi>, "Value"=w401:i16)  [unwired: 1 in, 1 out]
        n302 = call "数字键盘.vi"("OldNumber"=w401) -> ("NewNumber"=w400:sgl)
        n303 = property class="DigNum (严格)"(reference=w402, "Val(Sgnl)"=w400) -> ()  [unwired: 1 in, 2 out]
      }
      event "流量阈值": Mouse Down {
        n304 = event-data() -> ("CtlRef"=w407:refnum<vi>)  [unwired: 1 in, 7 out]
        n305 = property class="DigNum (严格)"(reference=w407) -> (reference out=w406:refnum<vi>, "Value"=w405:dbl)  [unwired: 1 in, 1 out]
        n306 = call "数字键盘.vi"("OldNumber"=w405) -> ("NewNumber"=w404:sgl)
        n307 = property class="DigNum (严格)"(reference=w406, "Val(Sgnl)"=w404) -> ()  [unwired: 1 in, 2 out]
      }
      event "时间阈值": Mouse Down {
        n308 = event-data() -> ("CtlRef"=w411:refnum<vi>)  [unwired: 1 in, 7 out]
        n309 = property class="DigNum (严格)"(reference=w411) -> (reference out=w410:refnum<vi>, "Value"=w409:u16)  [unwired: 1 in, 1 out]
        n310 = call "数字键盘.vi"("OldNumber"=w409) -> ("NewNumber"=w408:sgl)
        n311 = property class="DigNum (严格)"(reference=w410, "Val(Sgnl)"=w408) -> ()  [unwired: 1 in, 2 out]
      }
      event "开机启动": Value Change {
        n312 = event-data() -> ("NewVal"=w413:bool)  [unwired: 1 in, 5 out]
        n313 = call <vilib>:"Application Directory.vi"() -> ("Application Directory"=w412:path)
        n314 = case shown="假" w413 {
          tunnel: w412 -> [_ w418]
          frame False {
            n315 = call "删除启动项.vi"() -> ("删除标记"=w414:bool)  [unwired: 10 in, 1 out]
            n316 = case shown="假" w414 {
              frame False {
                n317 = local write "开机启动"(TRUE ("开机启动")) -> ()
                n318 = One Button Dialog(message="启动项删除失败" ("消息")) -> ()  [unwired: 1 in, 1 out]
              }
              frame True {
              }
            }
          }
          frame True {
            n319 = call "添加启动项.vi"("启动文件路径"=w418) -> ("添加成功标记"=w417:bool)  [unwired: 9 in, 1 out]
            n320 = case shown="假" w417 {
              frame False {
                n321 = local write "开机启动"(FALSE ("开机启动")) -> ()
                n322 = One Button Dialog(message="启动项添加失败" ("消息")) -> ()  [unwired: 1 in, 1 out]
              }
              frame True {
              }
            }
          }
        }
      }
      event "副屏显示设置": Value Change {
        n323 = event-data() -> ()  [unwired: 1 in, 6 out]
        n324 = call "副屏设置.vi"() -> ()  [unwired: 12 in]
      }
      event "首页显示设置": Value Change {
        n325 = event-data() -> ()  [unwired: 1 in, 6 out]
        n326 = call "首页显示设置.vi"() -> ()  [unwired: 12 in]
      }
      event "短信报警设置": Value Change {
        n327 = event-data() -> ()  [unwired: 1 in, 6 out]
        n328 = invoke class="VI" method="FP.Open"(reference=w423, "Activate"=TRUE ("激活？"), "State"=T7."Standard" ("状态")) -> ()  [unwired: 2 in, 5 out]
      }
      event "布尔": Mouse Down {
        n329 = event-data() -> ("CtlRef"=w425:refnum<vi>)  [unwired: 1 in, 7 out]
        n330 = property class="Bool (严格)"(reference=w425) -> ("Value"=w424:bool)  [unwired: 1 in, 2 out]
        n331 = case shown="假" w424 {
          tunnel: [w427 _] -> w426
          frame False {
            n332 = call "数字密码键盘.vi"() -> ("NewNumber"=w427:sgl)  [unwired: 1 in]
          }
          frame True {
          }
        }
        n333 = local write "输入密码"(w426) -> ()
      }
    }
  }
  n334 = local write "updateconfiguration"(w1) -> ()
  n335 = global write "update全局.vi" "updateconfiguration"(w1) -> ()
  n336 = while {
    tunnel: [w428] -> _
    tunnel: w15 -> [_]
    stop <- FALSE stop-if-true
    n337 = event shown="[0] 超时" {
      selector: _ -> [_ _ _]
      dyn-events: _ -> [_ _ _]
      timeout: 1000 -> [_ _ _]
      tunnel: [_ w439 _] -> w428
      event Timeout {
        n338 = event-data() -> ()  [unwired: 1 in, 3 out]
        n339 = local read "updateconfiguration"() -> (w431:T1)
        n340 = global write "update全局.vi" "updateconfiguration"(w431) -> ()
      }
      event "updateconfiguration": Value Change {
        n341 = event-data() -> ()  [unwired: 1 in, 6 out]
        n342 = Build Array("主机" ("section"), "用户" ("section"), "密码" ("key"), "远程路径" ("key"), "下载文件名" ("key"), "软件版本" ("key")) -> (w432:string[])
        n343 = call <vilib>:"Application Directory.vi"() -> ("Application Directory"=w442:path)
        n344 = Build Path(base path=w442, name or relative path="update\\data\\set.ini" ("名称或相对路径")) -> (appended path=w440:path)
        n345 = call "配置文件write.vi"("configuration file path"=w440, "键数组"=w432, "段"="应用程序交互" ("section")) -> ("error out"=w439:errorcluster)  [unwired: 8 in]
      }
      event "更新": Value Change {
        n346 = event-data() -> ()  [unwired: 1 in, 6 out]
        n347 = call "FTP自动升级更新main.vi"() -> ()  [unwired: 12 in]
      }
    }
  }
